vi "Dashboard Main.vi"() -> ()   [LabVIEW 2012]
uses:
  <vilib>/event_ctls.llb/eventvkey.ctl
  <vilib>/Utility/config.llb/Read Key (String).vi
  <vilib>/Utility/config.llb/Read Key (I32).vi
  <vilib>/Utility/config.llb/Write Key (String).vi
  <vilib>/Utility/config.llb/Write Key (I32).vi
  <vilib>/Utility/config.llb/NI_LVConfig.lvlib
panel:
  out "Climb Retical":bool
  out "Climb State":T1(ring)
  in  "ManualRPMPID":bool
  in  "ManualArmPID":bool
  in  "RPM PID gains":T2={"proportional gain (Kc)"=1.0, "integral time (Ti, min)"=0.01, "derivative time (Td, min)"=0.0} {"derivative time (Td, min)" format="%.3f"; "integral time (Ti, min)" format="%.3f"; "proportional gain (Kc)" format="%.3f"}
  in  "Arm PID gains":T2={"proportional gain (Kc)"=1.0, "integral time (Ti, min)"=0.01, "derivative time (Td, min)"=0.0} {"derivative time (Td, min)" format="%.3f"; "integral time (Ti, min)" format="%.3f"; "proportional gain (Kc)" format="%.3f"}
  out "Secondary":T3 {"Slide" scale=-1.0..1.0; "Trigger" scale=-1.0..1.0}
  out "Primary":T3 {"Slide" scale=-1.0..1.0; "Trigger" scale=-1.0..1.0}
  in  "stop? (T)":bool
  out "RPM":dbl(slide) scale=0.0..10.0
  out "Arm":T4
  out "Right":dbl(slide) scale=-1.0..1.0
  out "Left":dbl(slide) scale=-1.0..1.0
  out "Battery Value":dbl(slide) scale=0.0..14.0 scale format="%#_2e"
  out "Battery":sgl(graph)
  in  "Camera Settings":T5={"Frate Rate"=30, "Compression"=30, "Size"=1} {"Frate Rate" scale=1.0..30.0; "Size" items=["640x480", "320x240", "160x120"]}
  out "Mode":T6(ring)=enum."Auto Disabled"
  out "Camera IP":string
  out "Robot IP":string
  in  "Dashboard Tab":enum32{"Operation", "Test", "Checklist"}(tab)
  in  "Slider":dbl(slide) scale=0.0..100.0 scale format="%#_3g"
  in  "On/Off":bool caption="Solenoid"
  in  "Test Name":u16(ring) items=["Select the test to run...", "Example Test", "-------------------------------", "List of tests is built in robot code.", "Replace with your own automated tests."]
  in  "Test Tree":string(tree)
  in  "Motor":cluster{"Value":dbl, "Enable":bool} {"Value" scale=-1.0..1.0 scale format="%#_3g"}
  out "Progress":T7 {"Test Progress" scale=0.0..100.0}
  in  "Rev/Fwd":cluster{"Forward":bool, "Reverse":bool}
  in  "Ring":u16(ring) items=["Auto", "Fixed indoor", "Fixed outdoor 1", "Fixed outdoor 2", "Fixed fluorescent 1", "Fixed fluorescent 2", "Hold current"]
  in  "Listbox":i32(listbox)
  in  "Viewer":enum32{"Camera Image", "Variables"}(tab)
  out "Mbps":dbl format="%#.1g"
  in  "Enable":bool
  in  "DB Camera Config":bool
  out "Mbps":bool
  out "fps":dbl format="%#.1g"
  out "Image Error Message":string="Timeout in Camera Communications"
  out "Camera Image":T8(plugin-control)
  out "Tree":string(tree)
  # "Drive & Motors"
  # "Robot IP:"
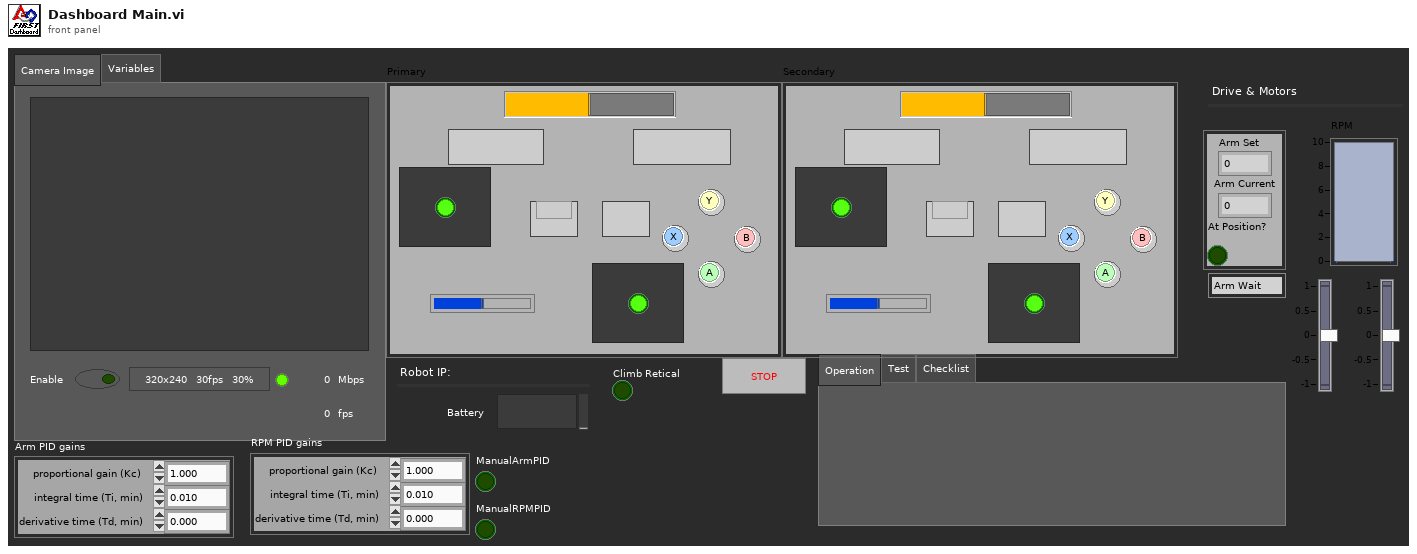
[diagram p1: front panel]
types:
  T1 = enum16{"Arm Wait", "Arm Up", "Arm Down", "Arm Attach"}
  T2 = cluster{"proportional gain (Kc)":dbl, "integral time (Ti, min)":dbl, "derivative time (Td, min)":dbl}
  T3 = cluster{"Y":bool, "B":bool, "X":bool, "A":bool, "Left Bumper":bool, "Right Bumper":bool, "Joystick 2":cluster{"X":dbl, "Y":dbl}[], "Joystick 3":cluster{"X":dbl, "Y":dbl}[], "Back":bool, "Start":bool, "Trigger":dbl, "Slide":dbl, "Right Thumbstick":bool, "Left Thumbstick":bool}
  T4 = cluster{"Arm Set":dbl, "Arm Current":dbl, "At Position?":bool}
  T5 = cluster{"Frate Rate":i32, "Compression":i32, "Size":u16}
  T6 = enum8{"Tele-Op Disabled", "Tele-Op Enabled", "Auto Disabled", "Auto Enabled", "Test Disabled", "Test Enabled", ""}
  T7 = cluster{"Test Progress":u8, "Test Progress Text":string}
  T8 = typedef "IMAQ Image.ctl" = refnum<image>
  T9 = typedef "Image Type" = u32
  T10 = typedef "LVRectTypeDef.ctl" = cluster{"Left":i16, "Top":i16, "Right":i16, "Bottom":i16}
  T11 = cluster{"Left":i32, "Top":i32, "Right":i32, "Bottom":i32}
  T12 = cluster{"Joy Stick":cluster{"Primary":cluster{"Buttons":cluster{"A":bool, "B":bool, "X":bool, "Y":bool, "Left Bumper":bool, "Right Bumper":bool, "Back":bool, "Start":bool, "Left Thumbstick":bool, "Right Thumbstick":bool}, "Axes":cluster{"Left Stick X ":dbl, "Left Stick Y":dbl, "Triggers":dbl, "Right Stick X":dbl, "Right Stick Y":dbl, "D-Pad X":dbl}}, "Secondary":cluster{"Buttons":cluster{"A":bool, "B":bool, "X":bool, "Y":bool, "Left Bumper":bool, "Right Bumper":bool, "Back":bool, "Start":bool, "Left Thumbstick":bool, "Right Thumbstick":bool}, "Axes":cluster{"Left Stick X ":dbl, "Left Stick Y":dbl, "Triggers":dbl, "Right Stick X":dbl, "Right Stick Y":dbl, "D-Pad X":dbl}}}, "Shooter":cluster{"RPM Current":dbl, "RPM Set":dbl, "In Range?":bool}, "Arm":cluster{"Arm Current":dbl, "Arm Set":dbl, "At Position?":bool}, "Drive":cluster{"Right":dbl, "Left":dbl}, "Climb State":enum16{"Arm Wait", "Arm Up", "Arm Down", "Arm Attach"}, "Change Retical":bool}
  T13 = cluster{"Arm PID gains":cluster{"proportional gain (Kc)":dbl, "integral time (Ti, min)":dbl, "derivative time (Td, min)":dbl}, "RPM PID gains":cluster{"proportional gain (Kc)":dbl, "integral time (Ti, min)":dbl, "derivative time (Td, min)":dbl}, "ManualArmPID?":bool, "ManualRPMPID?":bool, "EncodeReset":bool}
  T14 = cluster{"Competition mode":bool, "Robot Link":bool, "Autonomous":bool, "Enabled":bool, "E-Stop":bool, "Simulated":bool, "TestMode":bool, "Docked Window":bool}
  T15 = cluster{"Arm Current":dbl, "Arm Set":dbl, "At Position?":bool}
  T16 = cluster{"Buttons":cluster{"A":bool, "B":bool, "X":bool, "Y":bool, "Left Bumper":bool, "Right Bumper":bool, "Back":bool, "Start":bool, "Left Thumbstick":bool, "Right Thumbstick":bool}, "Axes":cluster{"Left Stick X ":dbl, "Left Stick Y":dbl, "Triggers":dbl, "Right Stick X":dbl, "Right Stick Y":dbl, "D-Pad X":dbl}}
  T17 = typedef "NI_LVConfig.lvlib/Config Data RefNum.ctl" = refnum<k1>
  T18 = typedef "eventvkey.ctl" = enum16{"ASCII", "Enter", "Return", "Shift", "Ctrl", "Alt", "Cmd", "Opt", "Caps", "NumLock", "Clear", "Break", "Up", "Down", "Left", "Right", "Insert", "Delete", "Home", "End", "PageUp", "PageDown", "Escape", "Help", "Pause", "ScrollLock", "F1", "F2", "F3", "F4", "F5", "F6", "F7", "F8", "F9", "F10", "F11", "F12", "F13", "F14", "F15", "F16", "F17", "F18", "F19", "F20", "F21", "F22", "F23", "F24", "Play", "VolumeUp", "VolumeDown", "Mute", "Two Byte Char"}
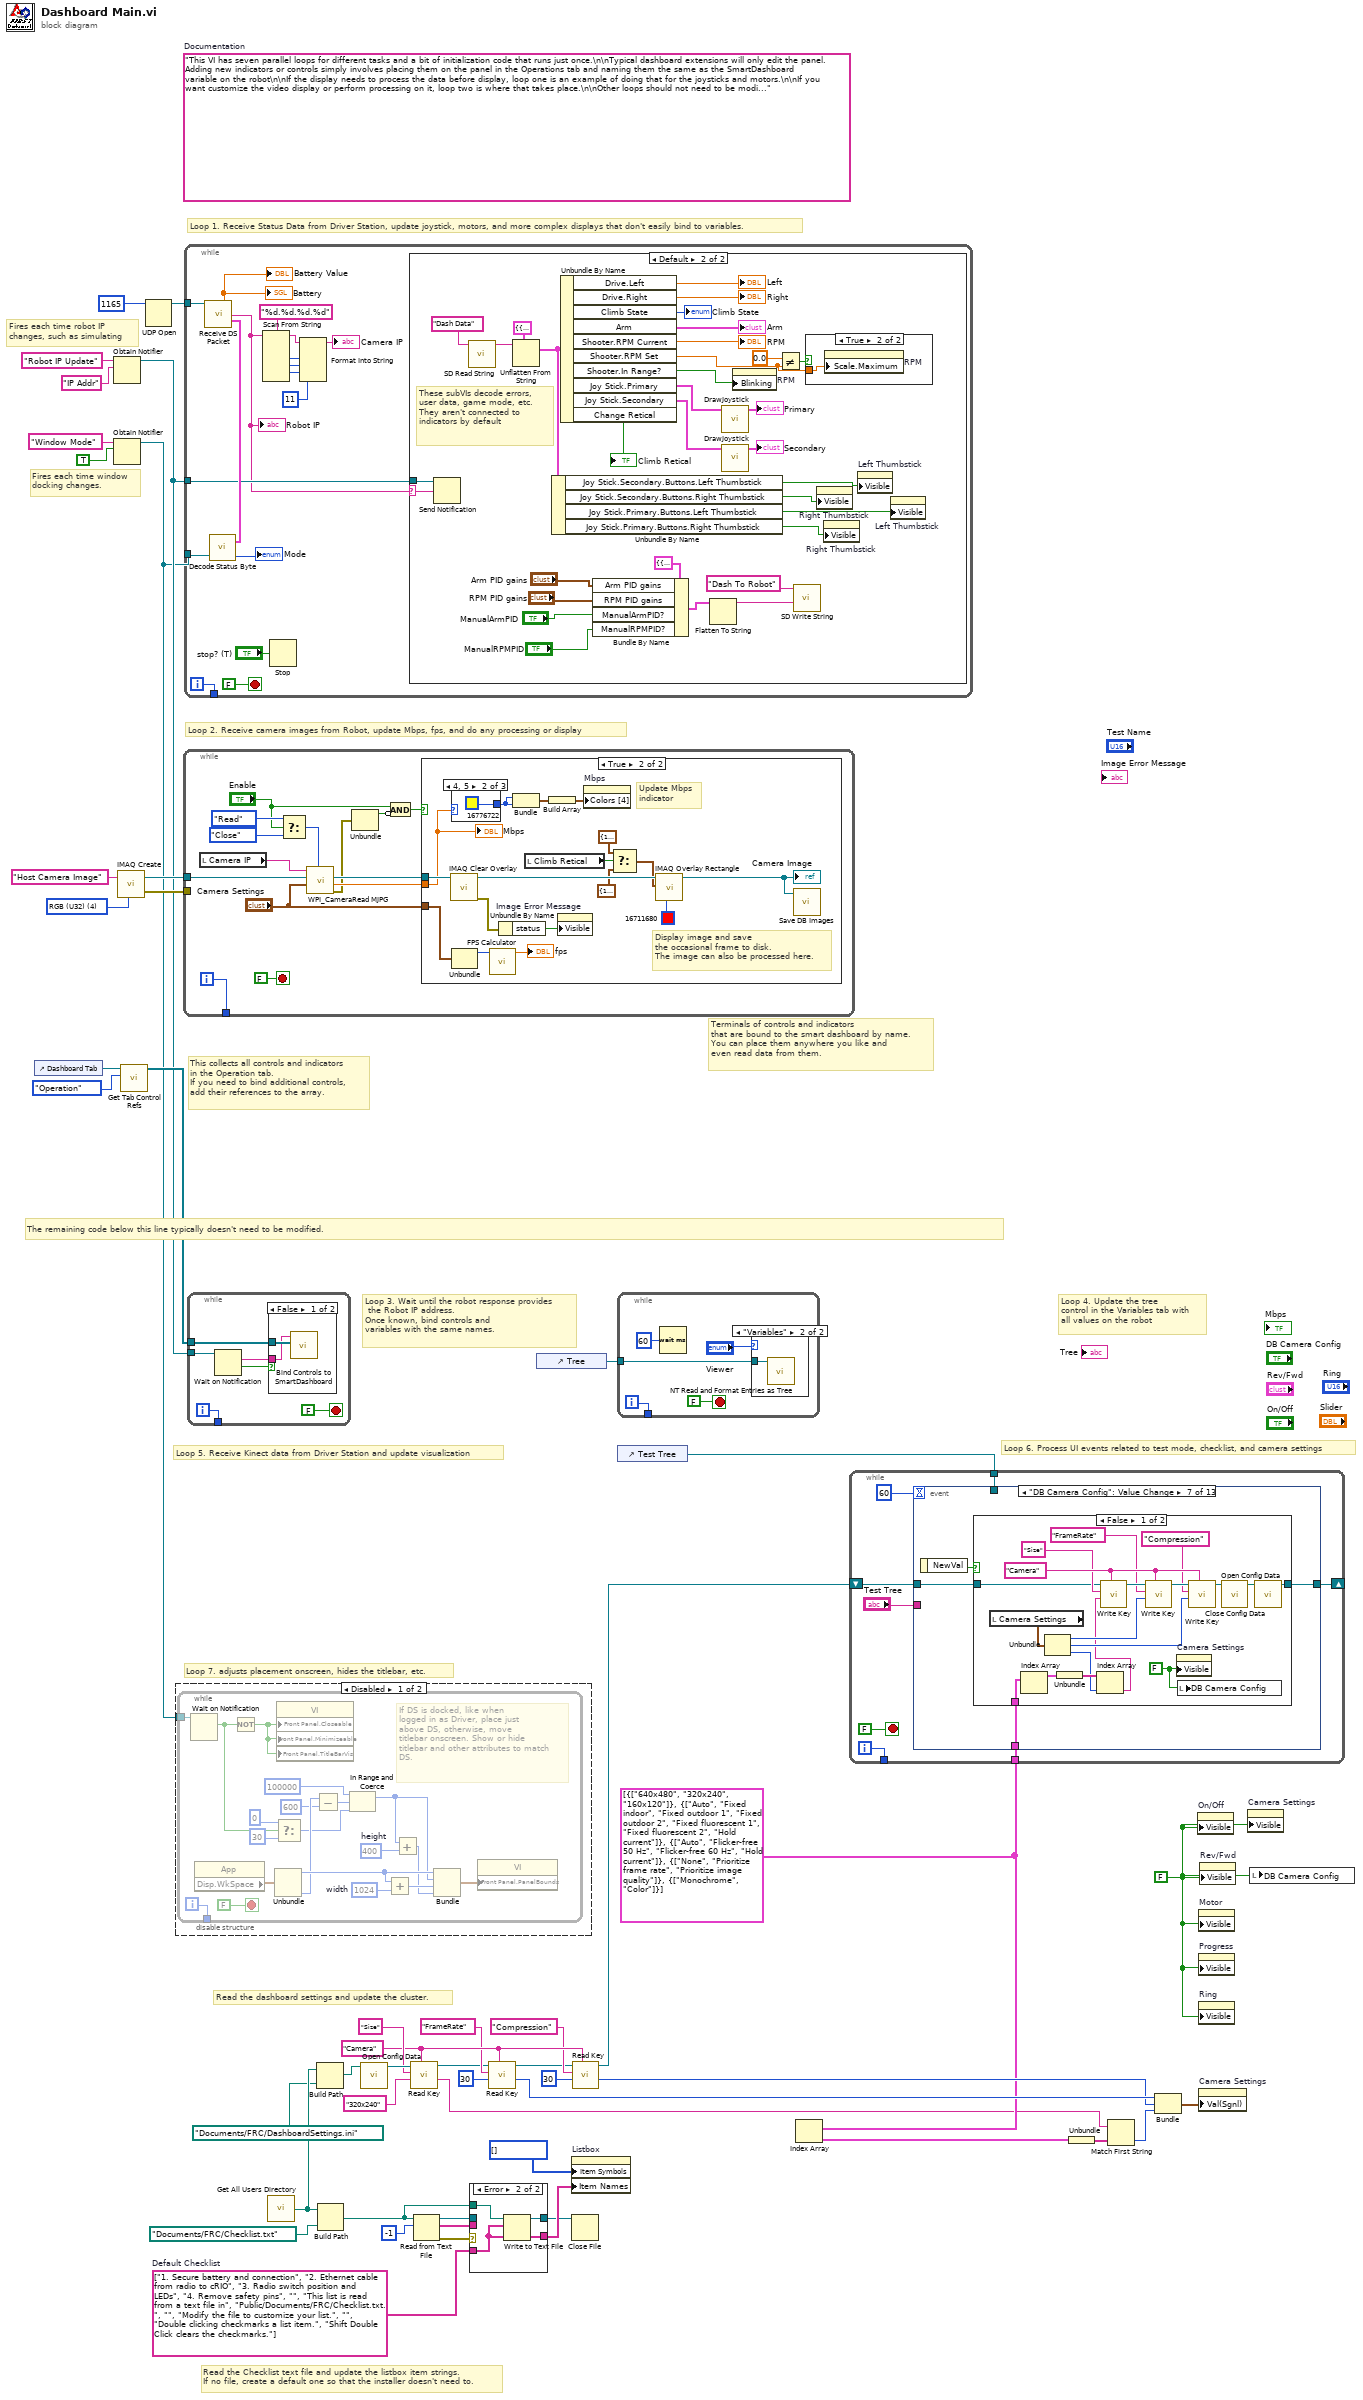
[diagram p0: block diagram]
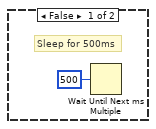
[diagram p4: hidden frame]
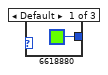
[diagram p5: hidden frame]
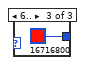
[diagram p6: hidden frame]
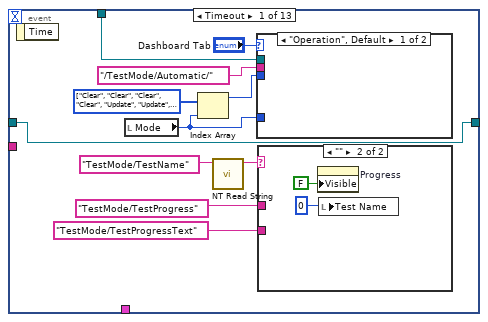
[diagram p8: hidden frame]
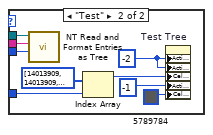
[diagram p9: hidden frame]
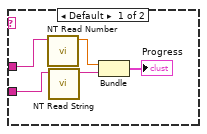
[diagram p10: hidden frame]
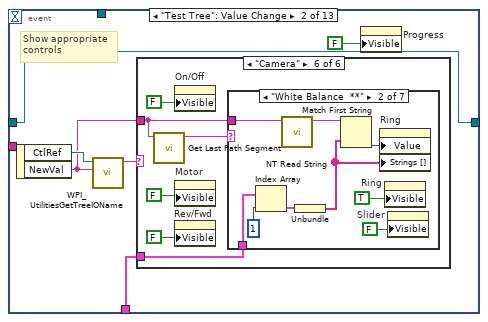
[diagram p11: hidden frame]
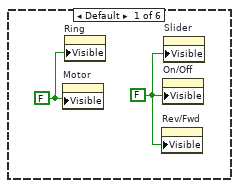
[diagram p12: hidden frame]
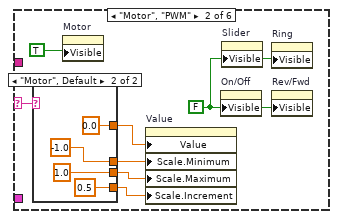
[diagram p13: hidden frame]
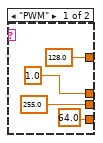
[diagram p14: hidden frame]
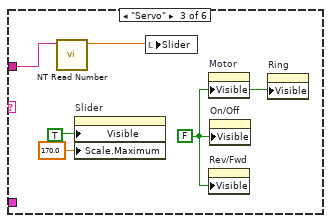
[diagram p15: hidden frame]
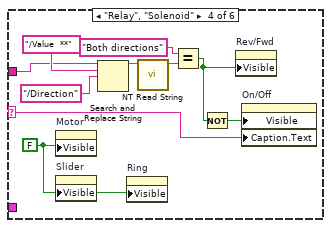
[diagram p16: hidden frame]
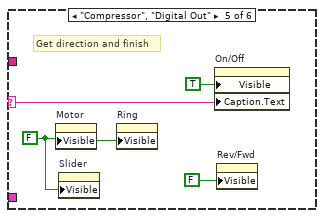
[diagram p17: hidden frame]
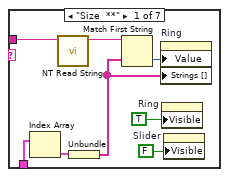
[diagram p18: hidden frame]
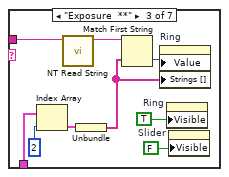
[diagram p19: hidden frame]
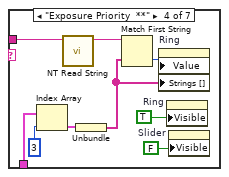
[diagram p20: hidden frame]
diagram:
  w21 = "Camera"
  w13 = cluster{string[]}[] [{["640x480", "320x240", "160x120"]}, {["Auto", "Fixed indoor", "Fixed outdoor 1", "Fixed outdoor 2", "Fixed fluorescent 1", "Fixed fluorescent 2", "Hold current"]}, {["Auto", "Flicker-free 50 Hz", "Flicker-free 60 Hz", "Hold current"]}, {["None", "Prioritize frame rate", "Prioritize image quality"]}, {["Monochrome", "Color"]}]
  w29 = string[] ["1. Secure battery and connection", "2. Ethernet cable from radio to cRIO", "3. Radio switch position and LEDs", "4. Remove safety pins", "", "This list is read from a text file in", "Public/Documents/FRC/Checklist.txt.", "", "Modify the file to customize your list.", "", "Double clicking checkmarks a list item.", "Shift Double Click clears the checkmarks."]  # Default Checklist
  w27 = FALSE ("Visible")
  (unwired) "This VI has seven parallel loops for different tasks and a bit of initialization code that runs just once.\n\nTypical dashboard extensions will only edit the panel. Adding new indicators or controls simply involves placing them on the panel in the Operations tab and naming them the same as the SmartDashboard variable on the robot\n\nIf the display needs to process the data before display, loop one is an example of doing that for the joysticks and motors.\n\nIf you want customize the video display or perform processing on it, loop two is where that takes place.\n\nOther loops should not need to be modified. They are pretty standard, and document the task they perform."  # Documentation
  w48 = T9 4 items=["Grayscale (U8)", "Grayscale (I16)", "Grayscale (SGL)", "Complex (CSG)", "RGB (U32)", "HSL (U32)", "RGB (U64)"] ("Image Type")
  # "Fires each time robot IP\nchanges, such as simulating"
  # "Fires each time window\ndocking changes."
  # "Read the Checklist text file and update the listbox item strings.\nIf no file, create a default one so that the installer doesn't need to."
  # "This collects all controls and indicators\nin the Operation tab.\nIf you need to bind additional controls,\nadd their references to the array."
  # "The remaining code below this line typically doesn't need to be modified."
  # "Loop 6. Process UI events related to test mode, checklist, and camera settings"
  # "Read the dashboard settings and update the cluster."
  # "Terminals of controls and indicators\nthat are bound to the smart dashboard by name.\nYou can place them anywhere you like and\neven read data from them."
  # "Loop 4. Update the tree\ncontrol in the Variables tab with\nall values on the robot"
  # "Loop 3. Wait until the robot response provides\n the Robot IP address.\nOnce known, bind controls and\nvariables with the same names."
  # "Loop 5. Receive Kinect data from Driver Station and update visualization"
  # "Loop 7. adjusts placement onscreen, hides the titlebar, etc."
  # "Loop 1. Receive Status Data from Driver Station, update joystick, motors, and more complex displays that don't easily bind to variables."
  # "Loop 2. Receive camera images from Robot, update Mbps, fps, and do any processing or display"
  n1 = control-ref of="Dashboard Tab"() -> (w43:refnum<vi>)
  n2 = Obtain Notifier(name (unnamed)="Robot IP Update", notification data type="IP Addr" ("name (unnamed)")) -> (notifier out=w40:refnum<notifier>)  [unwired: 2 in, 2 out]
  n3 = Obtain Notifier(name (unnamed)="Window Mode", notification data type=TRUE) -> (notifier out=w33:refnum<notifier>)  [unwired: 2 in, 2 out]
  n4 = call "IMAQ Create"("Image Name"="Host Camera Image", "Image Type"=w48) -> ("New Image"=w46:T8, "error out"=w45:errorcluster)  [unwired: 2 in, 1 out]
  n5 = call <vilib>:"Get Tab Control Refs.vi"("Page Index"=enum32{"Operation", "Test"}."Operation" ("Dashboard Tab"), "TabControl in"=w43) -> ("ControlsOnPage"=w44:refnum<vi>[])  [unwired: 9 in]
  n6 = UDP Open(11:u16 1165 ("port")) -> (port=w49:refnum<k16>)  [unwired: 2 in, 4 out]
  n7 = disable-structure shown="Disabled" {
    disable-tunnel: w33 -> [w51 _]
    frame Disabled {
      n8 = while {
        tunnel: w51 -> [w70]
        tunnel: [w68] -> _
        i -> [w68]
        stop <- FALSE stop-if-true
        w60 = 1024  # width
        w63 = 400  # height
        # "If DS is docked, like when\nlogged in as Driver, place just\nabove DS, otherwise, move\ntitlebar onscreen. Show or hide\ntitlebar and other attributes to match\nDS."
        n9 = Wait on Notification(notifier=w70) -> (notification=w55:bool)  [unwired: 3 in, 3 out]
        n10 = property class="App"() -> ("Disp.WkSpace"=w66:T10)  [unwired: 2 in, 2 out]
        n11 = Not(x=w55) -> (.not. x?=w69:bool)
        n12 = Unbundle(w66) -> ("Left"=w64:i16, "Bottom"=w61:i16)  [unwired: 2 out]
        n13 = Select(t=0, s=w55, f=30) -> (s? t:f=w54:i32)
        n14 = property class="VI"("Front Panel.Closeable"=w69, "Front Panel.Minimizeable"=w69, "Front Panel.TitleBarVis"=w69) -> ()  [unwired: 2 in, 2 out]
        n15 = Subtract(x=w61, y=600) -> (x-y=w58:i32)
        n16 = In Range and Coerce(upper limit=100000, x=w58, lower limit=w54) -> (coerced(x)=w52:i32)  [unwired: 1 out]
        n17 = Add(x=w64, y=w60) -> (x+y=w65:i32)
        n18 = Add(x=w52, y=w63) -> (x+y=w62:i32)
        n19 = Bundle("Left"=w64, w52, w65, w62) -> (w67:cluster{"Left":i16, i32, i32, i32})  [unwired: 1 out]
        n20 = property class="VI"("Front Panel.PanelBounds"=w67) -> ()  [unwired: 2 in, 2 out]
      }
    }
    frame Enabled {
    }
  }
  n21 = while {
    tunnel: w46 -> [w81]
    tunnel: w45 -> [_]
    tunnel: [w84] -> _
    i -> [w84]
    stop <- FALSE stop-if-true
    n22 = local read "Camera IP"() -> (w83:string)
    n23 = Select(t=enum16{"Read", "Reopen", "Close"}."Read" ("Operation"), s="Enable", f=enum16{"Read", "Reopen", "Close"}."Close" ("Operation")) -> (s? t:f=w76:enum16{"Read", "Reopen", "Close"})
    n24 = call <vilib>:"WPI_CameraRead MJPG.vi"("Operation"=w76, "Camera Settings"="Camera Settings", "Image"=w81, "address"=w83) -> ("error out"=w75:errorcluster, "Bandwidth (kbps)"=w79:dbl, "Image Out"=w80:T8)  [unwired: 5 in]
    n25 = Unbundle(w75) -> ("status"=w73:bool)  [unwired: 2 out]
    n26 = Compound Arithmetic op=AND("Enable", invert w73) -> (w72:bool)
    n27 = case shown="True" w72 {
      tunnel: "Camera Settings" -> [_ w95]
      tunnel: w80 -> [_ w98]
      tunnel: w79 -> [_ w97]
      frame False {
        # "Sleep for 500ms"
        n28 = Wait Until Next ms Multiple(millisecond multiple=u32 500) -> ()  [unwired: 1 out]
      }
      frame True {
        # "Display image and save\nthe occasional frame to disk.\nThe image can also be processed here."
        # "Update Mbps\nindicator"
        n29 = call "IMAQ Clear Overlay"("Image"=w98) -> ("error out"=w102:errorcluster, "Image Out"=w92:T8)  [unwired: 2 in, 7 out]
        n30 = case shown="4, 5" w97 {
          tunnel: [u32 6618880 ("Color Box") u32 16776722 ("Color Box") u32 16716800 ("Color Box")] -> w99
          frame Default {
          }
          frame 4, 5 {
          }
          frame 6.. {
          }
        }
        n31 = Unbundle(w95) -> ("Frate Rate"=w94:i32)  [unwired: 2 out]
        n32 = call "FPS Calculator.vi"("Average Count"=w94) -> ("fps"=→"fps":dbl)  [unwired: 10 in]
        n33 = Unbundle By Name(w102) -> ("status"=w103:bool)
        n34 = Bundle("Color Box"=w99, "Color Box"=w99) -> (w101:cluster{"Color Box":u32, "Color Box":u32})  [unwired: 1 out]
        n35 = local read "Climb Retical"() -> (w90:bool)
        n36 = Build Array(w101) -> (w100:cluster{"Color Box":u32, "Color Box":u32}[])
        n37 = property on="Image Error Message" class="Str"("Visible"=w103) -> ()  [unwired: 2 in, 2 out]
        n38 = property on="Mbps" class="Bool (strict)"("Colors [4]"=w100) -> ()  [unwired: 2 in, 2 out]
        n39 = Select(t=T11 {"Left"=10, "Top"=10, "Right"=1, "Bottom"=10}, s=w90, f=T11 {"Left"=10, "Top"=10, "Right"=10, "Bottom"=10} ("Rectangle")) -> (s? t:f=w89:T11)
        n40 = call "IMAQ Overlay Rectangle"("Color"=u32 16711680, "Rectangle"=w89, "Image"=w92) -> ("Image Out"=w91:T8)  [unwired: 7 in, 1 out]
        "Camera Image" <- w91
        n41 = call "Save DB Images.vi"("Image"=w91) -> ()  [unwired: 2 in, 1 out]
        "Mbps" <- w97
      }
    }
  }
  n42 = while {
    tunnel: w49 -> [w121]
    tunnel: w40 -> [w116]
    tunnel: w33 -> [w119]
    tunnel: [w117] -> _
    i -> [w117]
    stop <- FALSE stop-if-true
    n43 = call "Receive DS Packet.vi"("Recv Socket"=w121) -> ("Battery"=→"Battery" →"Battery Value":sgl, "Robot IP Address"=w110:string, "Status"=w122:T14)  [unwired: 1 in, 11 out]
    "Robot IP" <- w110
    n44 = call "Decode Status Byte.vi"("Window Mode Notifier"=w119, "Status"=w122) -> ("Mode"=→"Mode":T6)  [unwired: 1 out]
    n45 = Scan From String(format string="%d.%d.%d.%d", input string=w110) -> (remaining string=w108:string, output 1=w115:i32, output 2=w114:i32, output 3=w113:i32)  [unwired: 2 in, 7 out]
    n46 = Stop(stop? (T)="stop? (T)") -> ()
    n47 = Format Into String(initial string=w108, w115, w114, w113, 11 ("IP Suffix:")) -> (resulting string=→"Camera IP":string)  [unwired: 2 in, 1 out]
    n48 = case shown="Default" w110 {
      selector: w110 -> [_ w154]
      tunnel: w116 -> [_ w155]
      frame "0.0.0.0" {
        # "Robot not responding, don't poll the variables"
      }
      frame Default {
        # "These subVIs decode errors, user data, game mode, etc.\nThey aren't connected to indicators by default"
        n49 = Send Notification(notification=w154, notifier=w155) -> ()  [unwired: 1 in, 2 out]
        n50 = call <vilib>:"SD Read String.vi"("Name"="Dash Data") -> ("String"=w152:string)  [unwired: 8 in, 2 out]
        n51 = Unflatten From String(type=T12 {"Joy Stick"={"Primary"={"Buttons"={"A"=FALSE, "B"=FALSE, "X"=FALSE, "Y"=FALSE, "Left Bumper"=FALSE, "Right Bumper"=FALSE, "Back"=FALSE, "Start"=FALSE, "Left Thumbstick"=FALSE, "Right Thumbstick"=FALSE}, "Axes"={"Left Stick X "=0.0, "Left Stick Y"=0.0, "Triggers"=-0.0, "Right Stick X"=0.0, "Right Stick Y"=0.0, "D-Pad X"=0.0}}, "Secondary"={"Buttons"={"A"=FALSE, "B"=FALSE, "X"=FALSE, "Y"=FALSE, "Left Bumper"=FALSE, "Right Bumper"=FALSE, "Back"=FALSE, "Start"=FALSE, "Left Thumbstick"=FALSE, "Right Thumbstick"=FALSE}, "Axes"={"Left Stick X "=0.0, "Left Stick Y"=0.0, "Triggers"=0.0, "Right Stick X"=0.0, "Right Stick Y"=0.0, "D-Pad X"=0.0}}}, "Shooter"={"RPM Current"=0.0, "RPM Set"=0.0, "In Range?"=FALSE}, "Arm"={"Arm Current"=0.0, "Arm Set"=0.0, "At Position?"=FALSE}, "Drive"={"Right"=0.0, "Left"=0.0}, "Climb State"=enum."Arm Attach", "Change Retical"=FALSE} ("Dash Data"), binary string=w152) -> (value=w141:T12)  [unwired: 3 in, 2 out]
        n52 = Unbundle By Name(w141) -> ("Joy Stick.Secondary.Buttons.Left Thumbstick"=w138:bool, "Joy Stick.Secondary.Buttons.Right Thumbstick"=w137:bool, "Joy Stick.Primary.Buttons.Left Thumbstick"=w136:bool, "Joy Stick.Primary.Buttons.Right Thumbstick"=w135:bool)
        n53 = Unbundle By Name(w141) -> ("Drive.Left"=→"Left":dbl, "Drive.Right"=→"Right":dbl, "Climb State"=→"Climb State":T1, "Arm"=→"Arm":T15, "Shooter.RPM Current"=→"RPM":dbl, "Shooter.RPM Set"=w145:dbl, "Shooter.In Range?"=w147:bool, "Joy Stick.Primary"=w143:T16, "Joy Stick.Secondary"=w142:T16, "Change Retical"=→"Climb Retical":bool)
        n54 = Bundle By Name(cluster=T13 {"Arm PID gains"={"proportional gain (Kc)"=1.0, "integral time (Ti, min)"=0.01, "derivative time (Td, min)"=0.0}, "RPM PID gains"={"proportional gain (Kc)"=1.0, "integral time (Ti, min)"=0.01, "derivative time (Td, min)"=0.0}, "ManualArmPID?"=FALSE, "ManualRPMPID?"=FALSE, "EncodeReset"=FALSE} ("Dash to Robot"), "Arm PID gains"="Arm PID gains", "RPM PID gains"="RPM PID gains", "ManualArmPID?"="ManualArmPID", "ManualRPMPID?"="ManualRPMPID") -> (w129:T13)
        n55 = Flatten To String(anything=w129) -> (data string=w128:string)  [unwired: 3 in, 2 out]
        n56 = call "DrawJoystick.vi"("Joystick"=w143) -> ("DrawJoy"=→"Primary":T3)  [unwired: 10 in]
        n57 = call "DrawJoystick.vi"("Joystick"=w142) -> ("DrawJoy"=→"Secondary":T3)  [unwired: 10 in]
        n58 = property on="RPM" class="Slide (strict)"("Blinking"=w147) -> ()  [unwired: 2 in, 2 out]
        n59 = Not Equal?(x=0.0, y=w145) -> (x != y?=w146:bool)
        n60 = call <vilib>:"SD Write String.vi"("String"=w128, "Name"="Dash To Robot") -> ()  [unwired: 8 in, 2 out]
        n61 = case shown="True" w146 {
          tunnel: w145 -> [_ w156]
          frame False {
          }
          frame True {
            n62 = property on="RPM" class="Slide (strict)"("Scale.Maximum"=w156) -> ()  [unwired: 2 in, 2 out]
          }
        }
        n63 = property on="Right Thumbstick" class="Bool (strict)"("Visible"=w137) -> ()  [unwired: 2 in, 2 out]
        n64 = property on="Right Thumbstick" class="Bool (strict)"("Visible"=w135) -> ()  [unwired: 2 in, 2 out]
        n65 = property on="Left Thumbstick" class="Bool (strict)"("Visible"=w138) -> ()  [unwired: 2 in, 2 out]
        n66 = property on="Left Thumbstick" class="Bool (strict)"("Visible"=w136) -> ()  [unwired: 2 in, 2 out]
      }
    }
  }
  n67 = while {
    tunnel: w44 -> [w162]
    tunnel: w40 -> [w159]
    tunnel: [w157] -> _
    i -> [w157]
    stop <- FALSE stop-if-true
    n68 = Wait on Notification(notifier=w159) -> (notification=w158:string, timed out?=w160:bool)  [unwired: 3 in, 2 out]
    n69 = case shown="False" w160 {
      tunnel: w162 -> [w164 _]
      tunnel: w158 -> [w163 _]
      frame False {
        n70 = call <vilib>:"Bind Controls to SmartDashboard.vi"("Bound Control Refs"=w164, "Server IP Address"=w163) -> ()  [unwired: 10 in]
      }
      frame True {
      }
    }
  }
  n71 = call "Get All Users Directory.vi"() -> ("All User Path"=w26:path)
  n72 = Build Path(base path=w26, name or relative path=path "Documents/FRC/DashboardSettings.ini") -> (appended path=w25:path)
  n73 = Build Path(base path=w26, name or relative path=path "Documents/FRC/Checklist.txt") -> (appended path=w30:path)
  n74 = call <vilib>:"Open Config Data.vi"("configuration file path"=w25) -> ("refnum"=w24:T17)  [unwired: 8 in, 2 out]
  n75 = call-poly <vilib>:"Read Key.vi"("section"=w21, "default value"="320x240", "key"="Size", "refnum"=w24) -> ("value"=w11:string, "refnum out"=w6:T17)  [unwired: 2 in, 4 out]
  n76 = Read from Text File(file (use dialog)=w30, count=-1 ("timeout ms (25000)")) -> (refnum out=w8:refnum<file>, text=w31:string[], error out=w32:errorcluster)  [unwired: 2 in, 1 out]
  n77 = case shown="Error" w32 {
    tunnel: w31 -> [w166 _]
    tunnel: [w166 w168] -> w28
    tunnel: w29 -> [_ w168]
    tunnel: w30 -> [_ w169]
    tunnel: [w165 w167] -> w7
    tunnel: w8 -> [w165 _]
    frame No Error {
    }
    frame Error {
      n78 = Write to Text File(file (use dialog)=w169, text=w168) -> (refnum out=w167:refnum<file>)  [unwired: 2 in, 2 out]
    }
  }
  n79 = call-poly <vilib>:"Read Key.vi"("section"=w21, "default value"=30, "key"="FrameRate", "refnum"=w6) -> ("value"=w16:i32, "refnum out"=w5:T17)  [unwired: 1 in, 5 out]
  n80 = control-ref of="Tree"() -> (w2:refnum<vi>)
  n81 = property on="Listbox" class="LstBox (strict)"("Item Symbols"=i32[] [], "Item Names"=w28) -> ()  [unwired: 2 in, 2 out]
  n82 = Close File(refnum=w7) -> ()  [unwired: 1 in, 2 out]
  n83 = call-poly <vilib>:"Read Key.vi"("section"=w21, "default value"=30, "key"="Compression", "refnum"=w5) -> ("value"=w15:i32, "refnum out"=w3:T17)  [unwired: 1 in, 5 out]
  n84 = while {
    tunnel: [w171] -> _
    tunnel: w2 -> [w170]
    i -> [w171]
    stop <- FALSE stop-if-true
    n85 = Wait (ms)(milliseconds to wait=u32 60) -> ()  [unwired: 1 out]
    n86 = case shown="\"Variables\"" "Viewer" {
      tunnel: w170 -> [_ w175]
      frame Default {
      }
      frame "Variables" {
        n87 = call <vilib>:"NT Read and Format Entries as Tree.vi"("Tree Refnum"=w175) -> ()  [unwired: 9 in, 2 out]
      }
    }
  }
  n88 = control-ref of="Test Tree"() -> (w1:refnum<vi>)
  n89 = Index Array(array=w13) -> (element=w14:cluster{string[]})  [unwired: 1 in]
  n90 = while {
    tunnel: w13 -> [w180]
    shift-right: [w179] -> _
    shift-left: w3 -> [w178]
    tunnel: [w177] -> _
    tunnel: w1 -> [w176]
    i -> [w177]
    stop <- FALSE stop-if-true
    n91 = event shown="[6] \"DB Camera Config\": Value Change" {
      selector: _ -> [_ _ _ _ _ _ _ _ _ _ _ _ _]
      dyn-events: _ -> [_ _ _ _ _ _ _ _ _ _ _ _ _]
      timeout: u32 60 ("milliseconds to wait") -> [_ _ _ _ _ _ _ _ _ _ _ _ _]
      tunnel: w176 -> [w190 _ _ _ _ _ _ _ _ _ _ _ _]
      tunnel: "Test Tree" -> [_ _ _ _ _ _ _ _ w384 w392 w394 w398 w406]
      tunnel: w180 -> [_ w212 _ _ _ _ w348 w378 _ _ _ _ _]
      tunnel: [w184 w211 _ w314 w322 w334 w347 w371 w383 w390 w393 w397 w405] -> w179
      tunnel: w178 -> [w184 w211 _ w314 w322 w334 w346 w371 w383 w390 w393 w397 w405]
      event Timeout {
        w189 = enum16{"Update", "Clear"}[] [enum."Clear", enum."Clear", enum."Clear", enum."Clear", enum."Update", enum."Update", enum."Clear"] items=["Update", "Clear"]
        n92 = event-data() -> ()  [unwired: 1 in, 1 out]
        n93 = local read "Mode"() -> (w187:T6)
        n94 = Index Array(array=w189, index=w187) -> (element=w188:enum16{"Update", "Clear"})
        n95 = call <vilib>:"NT Read String.vi"("Name"="TestMode/TestName") -> ("String"=w193:string)  [unwired: 9 in, 1 out]
        n96 = case shown="\"Operation\", Default" "Dashboard Tab" {
          tunnel: w190 -> [_ w203]
          tunnel: "/TestMode/Automatic/" ("Name Pattern") -> [_ w202]
          tunnel: w188 -> [_ w201]
          tunnel: w187 -> [_ w199]
          frame "Operation", Default {
          }
          frame "Test" {
            w198 = -2 ("Active Item:Row Number")
            n97 = call <vilib>:"NT Read and Format Entries as Tree.vi"("Operation"=w201, "Name Pattern"=w202, "Tree Refnum"=w203) -> ()  [unwired: 7 in, 2 out]
            n98 = Index Array(array=u32[] [14013909, 14013909, 14013909, 14013909, 14013909, 16777215, 14013909], index=w199) -> (element=w197:u32)
            n99 = property on="Test Tree" class="Tree (strict)"("Active Item Row Number"=w198, "ActiveColNum"=w198, "CellBG"=w197, "Active Item Row Number"=-1 ("Active Item:Row Number"), "CellBG"=u32 5789784 ("Color Box")) -> ()  [unwired: 2 in, 2 out]
          }
        }
        n100 = case shown="\"\"" w193 {
          tunnel: "TestMode/TestProgress" ("Name") -> [w205 _]
          tunnel: "TestMode/TestProgressText" ("Name") -> [w204 _]
          frame Default {
            n101 = call <vilib>:"NT Read Number.vi"("Name"=w205) -> ("Numeric"=w206:dbl)  [unwired: 9 in, 1 out]
            n102 = call <vilib>:"NT Read String.vi"("Name"=w204) -> ("String"=w207:string)  [unwired: 9 in, 1 out]
            n103 = Bundle("Numeric"=w206, "String"=w207) -> (→"Progress":cluster{"Numeric":dbl, "String":string})  [unwired: 1 in]
          }
          frame "" {
            n104 = property on="Progress" class="Clust (strict)"("Visible"=FALSE) -> ()  [unwired: 2 in, 2 out]
            n105 = local write "Test Name"(u16 0) -> ()
          }
        }
      }
      event "Test Tree": Value Change {
        # "Show appropriate\ncontrols"
        n106 = event-data() -> ("CtlRef"=w215:refnum<vi>, "NewVal"=w213:string)  [unwired: 1 in]
        n107 = call <vilib>:"WPI_UtilitiesGetTreeIOName.vi"("NewVal"=w213, "TreeControl in"=w215) -> ("I/O Name"=w216:string)  [unwired: 9 in]
        n108 = case shown="\"Camera\"" w216 {
          selector: w216 -> [_ w223 _ w241 w250 _]
          tunnel: w213 -> [_ _ w238 w240 _ w257]
          tunnel: w212 -> [_ _ _ _ _ w256]
          frame Default {
            w218 = FALSE ("Visible")
            w217 = FALSE ("Visible")
            n109 = property on="Motor" class="Clust (strict)"("Visible"=w217) -> ()  [unwired: 2 in, 2 out]
            n110 = property on="Ring" class="Ring (strict)"("Visible"=w217) -> ()  [unwired: 2 in, 2 out]
            n111 = property on="Rev/Fwd" class="Clust (strict)"("Visible"=w218) -> ()  [unwired: 2 in, 2 out]
            n112 = property on="On/Off" class="Bool (strict)"("Visible"=w218) -> ()  [unwired: 2 in, 2 out]
            n113 = property on="Slider" class="Slide (strict)"("Visible"=w218) -> ()  [unwired: 2 in, 2 out]
          }
          frame "Motor", "PWM" {
            w224 = FALSE ("Visible")
            n114 = case shown="\"Motor\", Default" w223 {
              tunnel: [1.0 ("Value") -1.0 ("Value")] -> w222
              tunnel: [255.0 ("Value") 1.0 ("Value")] -> w221
              tunnel: [128.0 ("Value") 0.0 ("Value")] -> w220
              tunnel: [64.0 ("Value") 0.5 ("Value")] -> w219
              frame "PWM" {
              }
              frame "Motor", Default {
              }
            }
            n115 = property on="Motor" class="Clust (strict)"("Visible"=TRUE) -> ()  [unwired: 2 in, 2 out]
            n116 = property on="Value" class="Slide (strict)"("Value"=w220, "Scale.Minimum"=w222, "Scale.Maximum"=w221, "Scale.Increment"=w219) -> ()  [unwired: 2 in, 2 out]
            n117 = property on="On/Off" class="Bool (strict)"("Visible"=w224) -> ()  [unwired: 2 in, 2 out]
            n118 = property on="Slider" class="Slide (strict)"("Visible"=w224) -> ()  [unwired: 2 in, 2 out]
            n119 = property on="Ring" class="Ring (strict)"("Visible"=w224) -> ()  [unwired: 2 in, 2 out]
            n120 = property on="Rev/Fwd" class="Clust (strict)"("Visible"=w224) -> ()  [unwired: 2 in, 2 out]
          }
          frame "Servo" {
            w236 = FALSE ("Visible")
            n121 = call <vilib>:"NT Read Number.vi"("Name"=w238) -> ("Numeric"=w237:dbl)  [unwired: 9 in, 1 out]
            n122 = property on="Slider" class="Slide (strict)"("Visible"=TRUE, "Scale.Maximum"=170.0 ("Scale.Range:Maximum")) -> ()  [unwired: 2 in, 2 out]
            n123 = local write "Slider"(w237) -> ()
            n124 = property on="Motor" class="Clust (strict)"("Visible"=w236) -> ()  [unwired: 2 in, 2 out]
            n125 = property on="Rev/Fwd" class="Clust (strict)"("Visible"=w236) -> ()  [unwired: 2 in, 2 out]
            n126 = property on="On/Off" class="Bool (strict)"("Visible"=w236) -> ()  [unwired: 2 in, 2 out]
            n127 = property on="Ring" class="Ring (strict)"("Visible"=w236) -> ()  [unwired: 2 in, 2 out]
          }
          frame "Relay", "Solenoid" {
            w239 = FALSE ("Visible")
            n128 = property on="Motor" class="Clust (strict)"("Visible"=w239) -> ()  [unwired: 2 in, 2 out]
            n129 = property on="Slider" class="Slide (strict)"("Visible"=w239) -> ()  [unwired: 2 in, 2 out]
            n130 = Search and Replace String(input string=w240, search string="/Value  **", replace string="/Direction") -> (result string=w246:string)  [unwired: 5 in, 3 out]
            n131 = property on="Ring" class="Ring (strict)"("Visible"=w239) -> ()  [unwired: 2 in, 2 out]
            n132 = call <vilib>:"NT Read String.vi"("Name"=w246) -> ("String"=w244:string)  [unwired: 9 in, 1 out]
            n133 = Equal?(x="Both directions", y=w244) -> (x = y?=w242:bool)
            n134 = Not(x=w242) -> (.not. x?=w243:bool)
            n135 = property on="Rev/Fwd" class="Clust (strict)"("Visible"=w242) -> ()  [unwired: 2 in, 2 out]
            n136 = property on="On/Off" class="Bool (strict)"("Visible"=w243, "Caption.Text"=w241) -> ()  [unwired: 2 in, 2 out]
          }
          frame "Compressor", "Digital Out" {
            w249 = FALSE ("Visible")
            # "Get direction and finish"
            n137 = property on="Motor" class="Clust (strict)"("Visible"=w249) -> ()  [unwired: 2 in, 2 out]
            n138 = property on="Slider" class="Slide (strict)"("Visible"=w249) -> ()  [unwired: 2 in, 2 out]
            n139 = property on="Ring" class="Ring (strict)"("Visible"=w249) -> ()  [unwired: 2 in, 2 out]
            n140 = property on="On/Off" class="Bool (strict)"("Visible"=TRUE, "Caption.Text"=w250) -> ()  [unwired: 2 in, 2 out]
            n141 = property on="Rev/Fwd" class="Clust (strict)"("Visible"=FALSE) -> ()  [unwired: 2 in, 2 out]
          }
          frame "Camera" {
            n142 = call <vilib>:"Get Last Path Segment.vi"("String in"=w257) -> ("String out"=w258:string)  [unwired: 10 in]
            n143 = property on="On/Off" class="Bool (strict)"("Visible"=FALSE) -> ()  [unwired: 2 in, 2 out]
            n144 = property on="Motor" class="Clust (strict)"("Visible"=FALSE) -> ()  [unwired: 2 in, 2 out]
            n145 = property on="Rev/Fwd" class="Clust (strict)"("Visible"=FALSE) -> ()  [unwired: 2 in, 2 out]
            n146 = case shown="\"White Balance  **\"" w258 {
              tunnel: w257 -> [w264 w273 w282 w291 w300 _ w306]
              tunnel: w256 -> [w262 w270 w279 w288 w297 _ _]
              frame "Size  **" {
                n147 = Index Array(array=w262) -> (element=w261:cluster{string[]})  [unwired: 1 in]
                n148 = call <vilib>:"NT Read String.vi"("Name"=w264) -> ("String"=w263:string)  [unwired: 9 in, 1 out]
                n149 = Unbundle(w261) -> (w259:string[])
                n150 = Match First String(2:w259, 3:w263) -> (0:w260:i32)  [unwired: 1 out]
                n151 = property on="Ring" class="Ring (strict)"("Value"=w260, "Strings []"=w259) -> ()  [unwired: 2 in, 2 out]
                n152 = property on="Ring" class="Ring (strict)"("Visible"=TRUE) -> ()  [unwired: 2 in, 2 out]
                n153 = property on="Slider" class="Slide (strict)"("Visible"=FALSE) -> ()  [unwired: 2 in, 2 out]
              }
              frame "White Balance  **" {
                n154 = Index Array(array=w270, index=1) -> (element=w271:cluster{string[]})
                n155 = call <vilib>:"NT Read String.vi"("Name"=w273) -> ("String"=w272:string)  [unwired: 9 in, 1 out]
                n156 = Unbundle(w271) -> (w268:string[])
                n157 = Match First String(2:w268, 3:w272) -> (0:w267:i32)  [unwired: 1 out]
                n158 = property on="Ring" class="Ring (strict)"("Value"=w267, "Strings []"=w268) -> ()  [unwired: 2 in, 2 out]
                n159 = property on="Ring" class="Ring (strict)"("Visible"=TRUE) -> ()  [unwired: 2 in, 2 out]
                n160 = property on="Slider" class="Slide (strict)"("Visible"=FALSE) -> ()  [unwired: 2 in, 2 out]
              }
              frame "Exposure  **" {
                n161 = Index Array(array=w279, index=2) -> (element=w280:cluster{string[]})
                n162 = call <vilib>:"NT Read String.vi"("Name"=w282) -> ("String"=w281:string)  [unwired: 9 in, 1 out]
                n163 = Unbundle(w280) -> (w276:string[])
                n164 = Match First String(2:w276, 3:w281) -> (0:w277:i32)  [unwired: 1 out]
                n165 = property on="Ring" class="Ring (strict)"("Value"=w277, "Strings []"=w276) -> ()  [unwired: 2 in, 2 out]
                n166 = property on="Ring" class="Ring (strict)"("Visible"=TRUE) -> ()  [unwired: 2 in, 2 out]
                n167 = property on="Slider" class="Slide (strict)"("Visible"=FALSE) -> ()  [unwired: 2 in, 2 out]
              }
              frame "Exposure Priority  **" {
                n168 = Index Array(array=w288, index=3) -> (element=w289:cluster{string[]})
                n169 = call <vilib>:"NT Read String.vi"("Name"=w291) -> ("String"=w290:string)  [unwired: 9 in, 1 out]
                n170 = Unbundle(w289) -> (w285:string[])
                n171 = Match First String(2:w285, 3:w290) -> (0:w286:i32)  [unwired: 1 out]
                n172 = property on="Ring" class="Ring (strict)"("Value"=w286, "Strings []"=w285) -> ()  [unwired: 2 in, 2 out]
                n173 = property on="Ring" class="Ring (strict)"("Visible"=TRUE) -> ()  [unwired: 2 in, 2 out]
                n174 = property on="Slider" class="Slide (strict)"("Visible"=FALSE) -> ()  [unwired: 2 in, 2 out]
              }
              frame "Color Enable  **" {
                n175 = Index Array(array=w297, index=4) -> (element=w298:cluster{string[]})
                n176 = call <vilib>:"NT Read String.vi"("Name"=w300) -> ("String"=w299:string)  [unwired: 9 in, 1 out]
                n177 = Unbundle(w298) -> (w294:string[])
                n178 = Match First String(2:w294, 3:w299) -> (0:w295:i32)  [unwired: 1 out]
                n179 = property on="Ring" class="Ring (strict)"("Value"=w295, "Strings []"=w294) -> ()  [unwired: 2 in, 2 out]
                n180 = property on="Ring" class="Ring (strict)"("Visible"=TRUE) -> ()  [unwired: 2 in, 2 out]
                n181 = property on="Slider" class="Slide (strict)"("Visible"=FALSE) -> ()  [unwired: 2 in, 2 out]
              }
              frame Default {
                n182 = property on="Ring" class="Ring (strict)"("Visible"=FALSE) -> ()  [unwired: 2 in, 2 out]
                n183 = property on="Slider" class="Slide (strict)"("Visible"=FALSE) -> ()  [unwired: 2 in, 2 out]
              }
              frame "Brightness  **", "Color Level  **", "Compression  **", "FPS  **", "Sharpness  **" {
                n184 = call <vilib>:"NT Read Number.vi"("Name"=w306) -> ("Numeric"=w305:dbl)  [unwired: 9 in, 1 out]
                n185 = local write "Slider"(w305) -> ()
                n186 = property on="Slider" class="Slide (strict)"("Visible"=TRUE, "Scale.Maximum"=100.0 ("Scale.Range:Maximum")) -> ()  [unwired: 2 in, 2 out]
                n187 = property on="Ring" class="Ring (strict)"("Visible"=FALSE) -> ()  [unwired: 2 in, 2 out]
              }
            }
          }
        }
        n188 = property on="Progress" class="Clust (strict)"("Visible"=FALSE) -> ()  [unwired: 2 in, 2 out]
      }
      event "Test Name": Mouse Enter {
        # "Populate the ring with the list of tests"
        n189 = event-data() -> ()  [unwired: 1 in, 1 out]
        n190 = call <vilib>:"NT Read String Array.vi"("Name"="TestMode/TestList") -> ("String Array"=w313:string[])  [unwired: 9 in, 1 out]
        n191 = Build Array (concatenate)("Select the test to run...", w313) -> (w312:string[])
        n192 = property on="Test Name" class="Ring (strict)"("Strings []"=w312) -> ()  [unwired: 2 in, 2 out]
      }
      event "Test Name": Value Change {
        w315 = FALSE ("Visible")
        # "Tell the robot the test name to run"
        n193 = event-data() -> ("NewVal"=w319:u16)  [unwired: 1 in]
        n194 = property on="Test Name" class="Ring (strict)"() -> ("Strings []"=w320:string[])  [unwired: 2 in, 2 out]
        n195 = local write "Progress"(T7 {"Test Progress"=0, "Test Progress Text"=""} ("Progress")) -> ()
        n196 = Index Array(array=w320, index=w319) -> (element=w318:string)
        n197 = call <vilib>:"NT Write String.vi"("String"=w318, "Name"="TestMode/TestName") -> ()  [unwired: 9 in, 1 out]
        n198 = property on="Progress" class="Clust (strict)"("Visible"=TRUE) -> ()  [unwired: 2 in, 2 out]
        n199 = property on="Motor" class="Clust (strict)"("Visible"=w315) -> ()  [unwired: 2 in, 2 out]
        n200 = property on="Slider" class="Slide (strict)"("Visible"=w315) -> ()  [unwired: 2 in, 2 out]
        n201 = property on="On/Off" class="Bool (strict)"("Visible"=w315) -> ()  [unwired: 2 in, 2 out]
        n202 = property on="Rev/Fwd" class="Clust (strict)"("Visible"=w315) -> ()  [unwired: 2 in, 2 out]
        n203 = property on="Ring" class="Ring (strict)"("Visible"=w315) -> ()  [unwired: 2 in, 2 out]
      }
      event "Listbox": Double Click {
        n204 = event-data() -> ("PlatMods.Shift"=w323:bool, "Row"=w325:i32)  [unwired: 1 in]
        n205 = case shown="False" w323 {
          tunnel: w325 -> [w329 _]
          tunnel: 1 -> [w328 _]
          frame False {
            n206 = property on="Listbox" class="LstBox (strict)"() -> ("Item Symbols"=w327:i32[])  [unwired: 2 in, 2 out]
            n207 = Replace Array Subset(array=w327, new element=w328, index=w329) -> (w326:i32[])
            n208 = property on="Listbox" class="LstBox (strict)"("Item Symbols"=w326) -> ()  [unwired: 2 in, 2 out]
          }
          frame True {
            w330 = 0 ("Top Row")
            n209 = property on="Listbox" class="LstBox (strict)"() -> ("Number of Rows"=w332:u32)  [unwired: 2 in, 2 out]
            n210 = Initialize Array(0, w332) -> (w331:i32[])
            n211 = property on="Listbox" class="LstBox (strict)"("Top Row"=w330, "Value"=w330, "Item Symbols"=w331) -> ()  [unwired: 2 in, 2 out]
          }
        }
      }
      event "Listbox": Key Down {
        n212 = event-data() -> ("VKey"=w336:T18)  [unwired: 1 in]
        n213 = case shown="\"Left\", \"Right\"" w336 {
          selector: w336 -> [w341 _]
          tunnel: eventvkey."Left" ("VKey") -> [w339 _]
          frame "Left", "Right" {
            n214 = Equal?(x=w339, y=w341) -> (x = y?=w340:bool)
            n215 = Select(t=0, s=w340, f=1) -> (s? t:f=w342:i32)
            n216 = property on="Listbox" class="LstBox (strict)"() -> ("Item Symbols"=w345:i32[])  [unwired: 2 in, 2 out]
            n217 = Replace Array Subset(array=w345, new element=w342, index="Listbox") -> (w344:i32[])
            n218 = property on="Listbox" class="LstBox (strict)"("Item Symbols"=w344) -> ()  [unwired: 2 in, 2 out]
          }
          frame Default {
          }
        }
      }
      event "DB Camera Config": Value Change {
        n219 = event-data() -> ("NewVal"=w349:bool)  [unwired: 1 in]
        n220 = case shown="False" w349 {
          tunnel: w348 -> [w358 _]
          tunnel: [w351 w369] -> w347
          tunnel: w346 -> [w350 w369]
          frame False {
            w365 = "Camera"
            w368 = FALSE ("Visible")
            n221 = local read "Camera Settings"() -> (w357:T5)
            n222 = Index Array(array=w358) -> (element=w361:cluster{string[]})  [unwired: 1 in]
            n223 = Unbundle(w357) -> ("Frate Rate"=w356:i32, "Compression"=w355:i32, "Size"=w359:u16)
            n224 = Unbundle(w361) -> (w360:string[])
            n225 = Index Array(array=w360, index=w359) -> (element=w354:string)
            n226 = call-poly <vilib>:"Write Key.vi"("section"=w365, "value"=w354, "key"="Size", "refnum"=w350) -> ("refnum out"=w367:T17)  [unwired: 2 in, 5 out]
            n227 = call-poly <vilib>:"Write Key.vi"("section"=w365, "value"=w356, "key"="FrameRate", "refnum"=w367) -> ("refnum out"=w366:T17)  [unwired: 1 in, 6 out]
            n228 = property on="Camera Settings" class="Clust (strict)"("Visible"=w368) -> ()  [unwired: 2 in, 2 out]
            n229 = local write "DB Camera Config"(w368) -> ()
            n230 = call-poly <vilib>:"Write Key.vi"("section"=w365, "value"=w355, "key"="Compression", "refnum"=w366) -> ("refnum out"=w352:T17)  [unwired: 1 in, 6 out]
            n231 = call <vilib>:"Close Config Data.vi"("refnum"=w352) -> ("file path"=w353:path)  [unwired: 2 in, 8 out]
            n232 = call <vilib>:"Open Config Data.vi"("configuration file path"=w353) -> ("refnum"=w351:T17)  [unwired: 8 in, 2 out]
          }
          frame True {
            n233 = property on="Camera Settings" class="Clust (strict)"("Visible"=TRUE) -> ()  [unwired: 2 in, 2 out]
          }
        }
      }
      event "Camera Settings": Value Change {
        n234 = event-data() -> ("NewVal"=w382:T5)  [unwired: 1 in]
        n235 = Index Array(array=w378) -> (element=w377:cluster{string[]})  [unwired: 1 in]
        n236 = Unbundle(w382) -> ("Frate Rate"=w373:i32, "Compression"=w372:i32, "Size"=w375:u16)
        n237 = Unbundle(w377) -> (w376:string[])
        n238 = Index Array(array=w376, index=w375) -> (element=w374:string)
        n239 = Format Into String(format string="%s   %dfps   %d%%", w374, w373, w372) -> (resulting string=w379:string)  [unwired: 2 in, 1 out]
        n240 = Build Array(w379) -> (w380:string[])
        n241 = property on="DB Camera Config" class="Bool (strict)"("Strings [4]"=w380) -> ()  [unwired: 2 in, 2 out]
      }
      event "Motor.Enable": Value Change {
        n242 = event-data() -> ("NewVal"=w388:bool)  [unwired: 1 in]
        n243 = Unbundle("Motor") -> ("Value"=w387:dbl)  [unwired: 1 out]
        n244 = Select(t=w387, s=w388, f=0.0) -> (s? t:f=w385:dbl)
        n245 = call <vilib>:"NT Write Number.vi"("Numeric"=w385, "Name"=w384) -> ()  [unwired: 9 in, 1 out]
      }
      event "Slider": Value Change {
        n246 = event-data() -> ("NewVal"=w391:dbl)  [unwired: 1 in]
        n247 = call <vilib>:"NT Write Number.vi"("Numeric"=w391, "Name"=w392) -> ()  [unwired: 9 in, 1 out]
      }
      event "On/Off": Value Change {
        n248 = event-data() -> ("NewVal"=w396:bool)  [unwired: 1 in]
        n249 = Boolean To (0,1)(Boolean=w396) -> (0, 1=w395:i16)
        n250 = call <vilib>:"NT Write Number.vi"("Numeric"=w395, "Name"=w394) -> ()  [unwired: 9 in, 1 out]
      }
      event "Rev/Fwd": Value Change {
        n251 = event-data() -> ("NewVal.Forward"=w404:bool, "NewVal.Reverse"=w403:bool)  [unwired: 1 in]
        n252 = Boolean To (0,1)(Boolean=w404) -> (0, 1=w400:i16)
        n253 = Boolean To (0,1)(Boolean=w403) -> (0, 1=w402:i16)
        n254 = Negate(x=w402) -> (-x=w401:i16)
        n255 = Add(x=w400, y=w401) -> (x+y=w399:i16)
        n256 = call <vilib>:"NT Write Number.vi"("Numeric"=w399, "Name"=w398) -> ()  [unwired: 9 in, 1 out]
      }
      event "Ring": Value Change {
        n257 = event-data() -> ("NewVal"=w408:u16)  [unwired: 1 in]
        n258 = property on="Ring" class="Ring (strict)"() -> ("Strings []"=w409:string[])  [unwired: 2 in, 2 out]
        n259 = Index Array(array=w409, index=w408) -> (element=w407:string)
        n260 = call <vilib>:"NT Write String.vi"("String"=w407, "Name"=w406) -> ()  [unwired: 9 in, 1 out]
      }
    }
  }
  n261 = Unbundle(w14) -> (w12:string[])
  n262 = Match First String(2:w12, 3:w11) -> (0:w10:i32)  [unwired: 1 out]
  n263 = Bundle("value"=w16, "value"=w15, "index"=w10) -> (w4:cluster{"value":i32, "value":i32, "index":i32})  [unwired: 1 out]
  n264 = property on="On/Off" class="Bool (strict)"("Visible"=w27) -> ()  [unwired: 2 in, 2 out]
  n265 = property on="Motor" class="Clust (strict)"("Visible"=w27) -> ()  [unwired: 2 in, 2 out]
  n266 = property on="Progress" class="Clust (strict)"("Visible"=w27) -> ()  [unwired: 2 in, 2 out]
  n267 = property on="Ring" class="Ring (strict)"("Visible"=w27) -> ()  [unwired: 2 in, 2 out]
  n268 = property on="Camera Settings" class="Clust (strict)"("Val(Sgnl)"=w4) -> ()  [unwired: 2 in, 2 out]
  n269 = property on="Rev/Fwd" class="Clust (strict)"("Visible"=w27) -> ()  [unwired: 2 in, 2 out]
  n270 = property on="Camera Settings" class="Clust (strict)"("Visible"=w27) -> ()  [unwired: 2 in, 2 out]
  n271 = local write "DB Camera Config"(w27) -> ()
